vi "initialize Session Data.vi"(0 "Session in":refnum<class "Test Number and Bin Generator.lvclass">=refnum, 11 "error in":errorcluster) -> (4 "Session out":refnum<class "Test Number and Bin Generator.lvclass">, 15 "error out":errorcluster)   [LabVIEW 2018, in "Test Number and Bin Generator.lvlib" / "Test Number and Bin Generator.lvclass"]
uses:
  Test Number and Bin Generator.lvclass
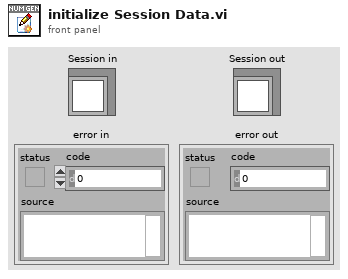
[diagram p1: front panel]
types:
  T1 = typedef "TestStand API Tools (TSAT).lvlibp/TSAT Evaluation Actions.lvlib/TSAT Evaluation.ctl" = cluster{"Test Name":string, "Pin":string, "Units":string, "SI Scaling":T2, "Test Number":i32, "Published Data Id":string, "Low Limit":dbl, "High Limit":dbl, "Export Data Location":string, "Software Bin":i64, "Evaluation Type":T3, "Test Data Source":string}
  T2 = typedef "TestStand API Tools (TSAT).lvlibp/TSAT Evaluation Actions.lvlib/TSAT Eval SI Unit Scaling.ctl" = i16
  T3 = typedef "TestStand API Tools (TSAT).lvlibp/TSAT Evaluation Actions.lvlib/TSAT Evaluation Type.ctl" = enum16{"Numeric Limit", "Pass/Fail", "None"}
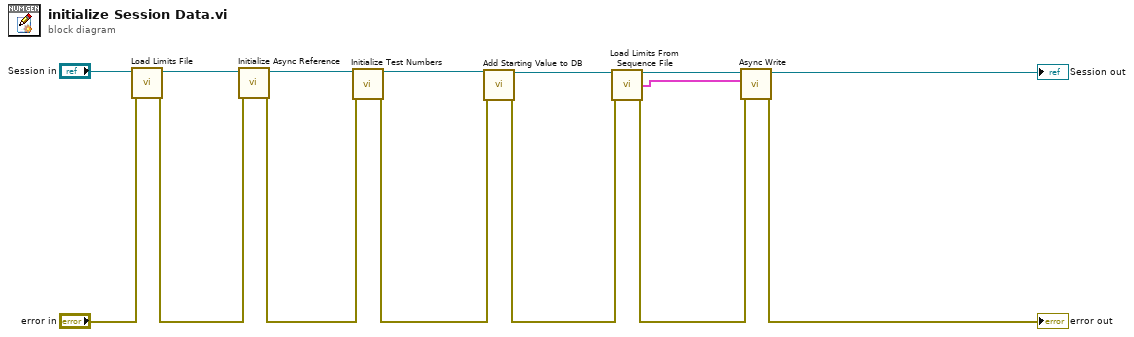
[diagram p0: block diagram]
diagram:
  n1 = call "Load Limits File.vi"("error in (no error)"="error in", "Test Number and Bin Generator In"="Session in") -> ("error out"=w13:errorcluster, "Test Number and Bin Generator Out"=w7:refnum<class "Test Number and Bin Generator.lvclass">)  [unwired: 8 in]
  n2 = call "Initialize Async Reference.vi"("error in (no error)"=w13, "Test Number and Bin Generator in"=w7) -> ("error out"=w5:errorcluster, "Test Number and Bin Generator out"=w6:refnum<class "Test Number and Bin Generator.lvclass">)  [unwired: 8 in]
  n3 = call "Initialize Test Numbers.vi"("Test Num and Bin Gen In"=w6, "error in (no error)"=w5) -> ("Test Num and Bin Gen Out"=w12:refnum<class "Test Number and Bin Generator.lvclass">, "error out"=w11:errorcluster)  [unwired: 12 in]
  n4 = call "Add Starting Value to DB.vi"("Test Number and Bin Generator In"=w12, "error in (no error)"=w11) -> ("Test Number and Bin Generator Out"=w3:refnum<class "Test Number and Bin Generator.lvclass">, "error out"=w10:errorcluster)  [unwired: 12 in]
  n5 = call "Load Limits From Sequence File.vi"("Test Number and Bin Generator"=w3, "error in (no error)"=w10) -> ("Test Number and Bin Generator 2"=w2:refnum<class "Test Number and Bin Generator.lvclass">, "Evaluations From Sequence File"=w1:T1[], "error out"=w4:errorcluster)  [unwired: 11 in]
  n6 = call "Async Write.vi"("error in (no error)"=w4, "Evaluations In"=w1, "Test Number and Bin Generator in"=w2) -> ("error out"=→"error out":errorcluster, "Test Number and Bin Generator out"=→"Session out":refnum<class "Test Number and Bin Generator.lvclass">)  [unwired: 7 in]
